vi "reaction_game.vi"() -> ()   [LabVIEW 2017]
panel:
  in  "stop":bool
  in  "Push Button":bool
  out "Result":dbl
  out "Message":string
  out "Indicator":bool
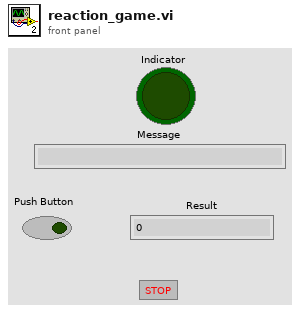
[diagram p1: front panel]
types:
  T1 = enum16{"Begin Game", "Random Wait", "Wait For Reaction", "Calculate Result"}
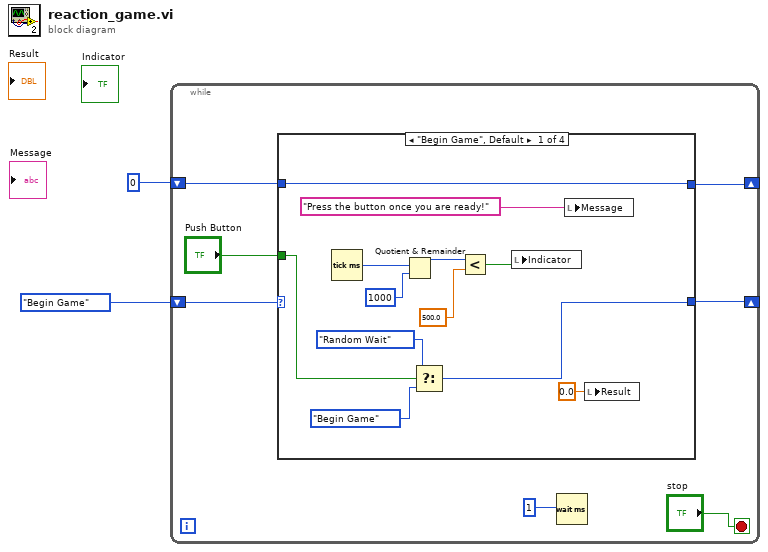
[diagram p0: block diagram]
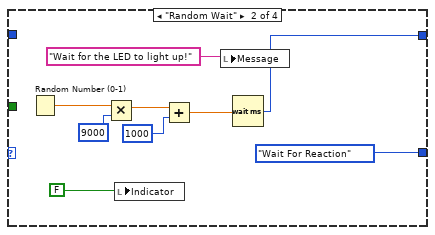
[diagram p2: hidden frame]
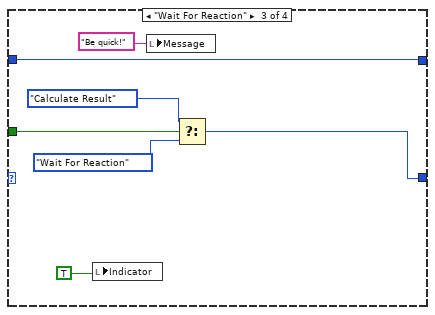
[diagram p3: hidden frame]
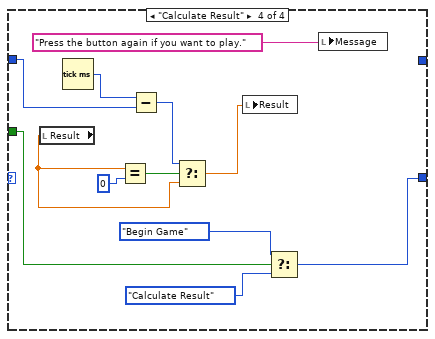
[diagram p4: hidden frame]
diagram:
  n1 = while {
    shift-right: [w6] -> _
    shift-left: T1."Begin Game" -> [w7]
    shift-right: [w4] -> _
    shift-left: 0 -> [w3]
    stop <- "stop" stop-if-true
    n2 = case shown="\"Begin Game\", Default" w7 {
      tunnel: "Push Button" -> [w15 _ w34 w40]
      tunnel: [w12 T1."Wait For Reaction" w31 w39] -> w6
      tunnel: [w11 w22 w37 _] -> w4
      tunnel: w3 -> [w11 _ w37 w48]
      frame "Begin Game", Default {
        n3 = Tick Count (ms)() -> (millisecond timer value=w20:u32)
        n4 = Quotient & Remainder(x=w20, y=1000) -> (x-y*floor(x/y)=w17:u32)  [unwired: 1 out]
        n5 = Select(t=T1."Random Wait", s=w15, f=T1."Begin Game") -> (s? t:f=w12:T1)
        n6 = Less?(x=w17, y=500.0) -> (x < y?=w16:bool)
        n7 = local write "Indicator"(w16) -> ()
        n8 = local write "Message"("Press the button once you are ready!") -> ()
        n9 = local write "Result"(0.0 ("Result")) -> ()
      }
      frame "Random Wait" {
        n10 = Random Number (0-1)() -> (number: 0 to 1=w28:dbl)
        n11 = Multiply(x=w28, y=9000) -> (x*y=w27:dbl)
        n12 = local write "Indicator"(FALSE) -> ()
        n13 = Add(x=w27, y=1000) -> (x+y=w26:dbl)
        n14 = local write "Message"("Wait for the LED to light up!") -> ()
        n15 = Wait (ms)(milliseconds to wait=w26) -> (millisecond timer value=w22:u32)
      }
      frame "Wait For Reaction" {
        n16 = local write "Indicator"(TRUE) -> ()
        n17 = local write "Message"("Be quick!") -> ()
        n18 = Select(t=T1."Calculate Result", s=w34, f=T1."Wait For Reaction") -> (s? t:f=w31:T1)
      }
      frame "Calculate Result" {
        n19 = local read "Result"() -> (w43:dbl)
        n20 = Tick Count (ms)() -> (millisecond timer value=w49:u32)
        n21 = Equal?(x=w43, y=0) -> (x = y?=w46:bool)
        n22 = Subtract(x=w49, y=w48) -> (x-y=w45:u32)
        n23 = Select(t=w45, s=w46, f=w43) -> (s? t:f=w47:dbl)
        n24 = local write "Result"(w47) -> ()
        n25 = Select(t=T1."Begin Game", s=w40, f=T1."Calculate Result") -> (s? t:f=w39:T1)
        n26 = local write "Message"("Press the button again if you want to play.") -> ()
      }
    }
    n27 = Wait (ms)(milliseconds to wait=1) -> ()  [unwired: 1 out]
  }
